vi "Meas Proc QWTB Set Result Table Sizes.vi"(7 "param table ref":refnum<vi>, 8 "error in":errorcluster) -> (0 "error out":errorcluster)   [LabVIEW 2020]
doc: "Sets widths of the table columns. This VI will identify which tables column width was modified and sets the same width to all other columns (except header)."
uses:
  <vilib>/Utility/miscctls.llb/LVRowAndColumnTypeDef.ctl
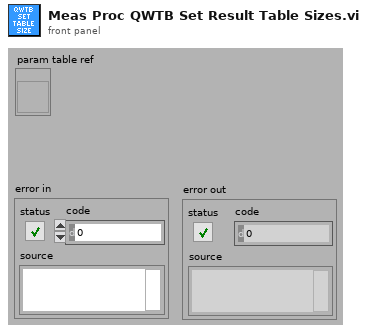
[diagram p1: front panel]
types:
  T1 = typedef "LVRowAndColumnTypeDef.ctl" = cluster{"Row":i32, "Column":i32}
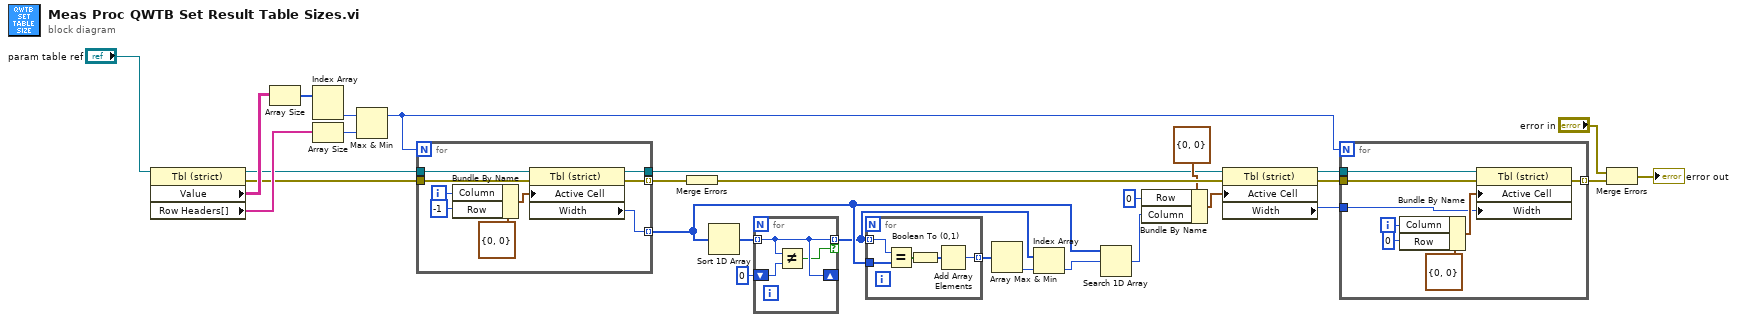
[diagram p0: block diagram]
diagram:
  n1 = property class="Tbl (strict)"(reference="param table ref") -> (reference out=w22:refnum<vi>, error out=w21:errorcluster, "Value"=w27:string[][], "Row Headers[]"=w24:string[])  [unwired: 1 in]
  n2 = Array Size(array=w27) -> (size(s)=w26:i32[])
  n3 = Index Array(array=w26) -> (element #2=w25:i32)  [unwired: 2 in, 1 out]
  n4 = Array Size(array=w24) -> (size(s)=w23:i32)
  n5 = Max & Min(x=w25, y=w23) -> (max(x,y)=w6:i32)  [unwired: 1 out]
  n6 = for {
    N: w6 -> [_]
    tunnel: w21 -> [w38]
    tunnel: [w33] -> w20 mode=indexing
    tunnel: w22 -> [w32]
    tunnel: [w31] -> w13
    tunnel: [w30] -> w5 mode=indexing
    i -> [w34]
    n7 = Bundle By Name(cluster=T1 {"Row"=0, "Column"=0} ("Active Cell:Active Cell"), "Column"=w34, "Row"=-1 ("Column")) -> (w37:T1)
    n8 = property class="Tbl (strict)"(reference=w32, error in=w38, "Active Cell"=w37) -> (reference out=w31:refnum<vi>, error out=w33:errorcluster, "Width"=w30:u32)
  }
  n9 = Merge Errors(w20) -> (w16:errorcluster)
  n10 = Sort 1D Array(array=w5) -> (sorted array=w18:u32[])
  n11 = for {
    tunnel: w18 -> [w40] mode=indexing
    shift-right: [w40] -> _
    shift-left: u32 0 -> [w41]
    tunnel: [w40] -> w2 mode=indexing if=w39
    n12 = Not Equal?(x=w40, y=w41) -> (x != y?=w39:bool)
  }
  n13 = for {
    tunnel: w2 -> [w46] mode=indexing
    tunnel: w5 -> [w45]
    tunnel: [w42] -> w17 mode=indexing
    n14 = Equal?(x=w46, y=w45) -> (x = y?=w44:bool[])
    n15 = Boolean To (0,1)(Boolean=w44) -> (0, 1=w43:i16[])
    n16 = Add Array Elements(numeric array=w43) -> (sum=w42:i16)
  }
  n17 = Array Max & Min(array=w17) -> (min index (indices)=w3:i32)  [unwired: 3 out]
  n18 = Index Array(array=w2, index=w3) -> (element=w1:u32)
  n19 = Search 1D Array(1D array=w5, element=w1) -> (index of element=w4:i32)  [unwired: 1 in]
  n20 = Bundle By Name(cluster=T1 {"Row"=0, "Column"=0} ("Active Cell:Active Cell"), "Row"=0, "Column"=w4) -> (w14:T1)
  n21 = property class="Tbl (strict)"(reference=w13, error in=w16, "Active Cell"=w14) -> (reference out=w10:refnum<vi>, error out=w11:errorcluster, "Width"=w9:u32)
  n22 = for {
    N: w6 -> [_]
    tunnel: w11 -> [w54]
    tunnel: w10 -> [w49]
    tunnel: w9 -> [w48]
    tunnel: [w47] -> w8 mode=indexing
    i -> [w50]
    n23 = Bundle By Name(cluster=T1 {"Row"=0, "Column"=0} ("Active Cell:Active Cell"), "Column"=w50, "Row"=0 ("Column")) -> (w53:T1)
    n24 = property class="Tbl (strict)"(reference=w49, error in=w54, "Active Cell"=w53, "Width"=w48) -> (error out=w47:errorcluster)  [unwired: 1 out]
  }
  n25 = Merge Errors("error in", w8) -> (→"error out":errorcluster)
